vi "Poll FP Change Device List.vi"(8 "Error In":errorcluster, 10 "First call?":bool, 11 "Device List State":T1) -> (0 "Error Out":errorcluster, 3 "Device List State out":T1)   [LabVIEW 2015]
uses:
  Device List State.ctl
  Device/Device.lvclass
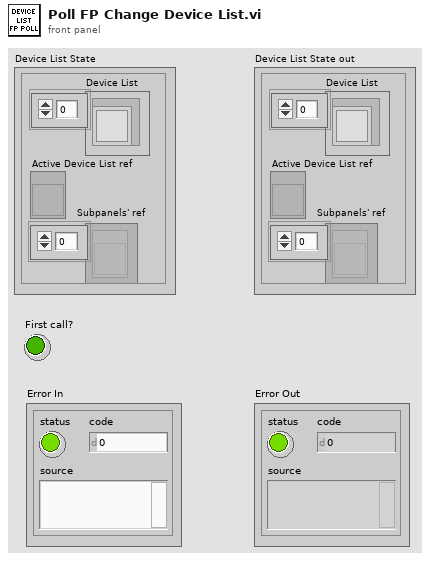
[diagram p1: front panel]
types:
  T1 = typedef "Device List State.ctl" = cluster{"Device List":refnum<class "Device.lvclass">[], "Active Device List ref":refnum<vi>, "Subpanels' ref":refnum<vi>[]}
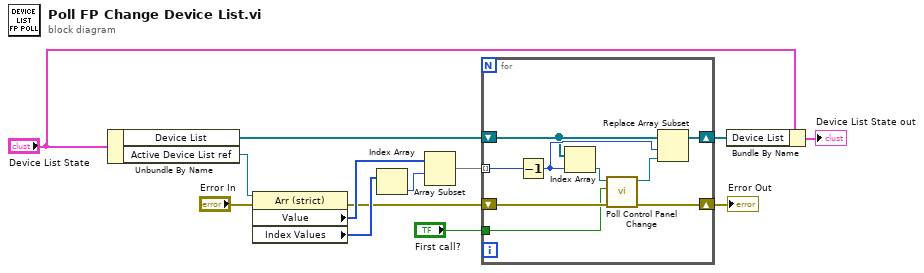
[diagram p0: block diagram]
diagram:
  n1 = Unbundle By Name("Device List State") -> ("Device List"=w7:refnum<class "Device.lvclass">[], "Active Device List ref"=w12:refnum<vi>)
  n2 = property class="Arr (strict)"(reference=w12, error in="Error In") -> (error out=w6:errorcluster, "Value"=w11:u16[], "Index Values"=w9:u32[])  [unwired: 1 out]
  n3 = Index Array(array=w9) -> (element=w10:u32)  [unwired: 1 in]
  n4 = Array Subset(array=w11, index=w10) -> (w8:u16[])  [unwired: 1 in]
  n5 = for {
    tunnel: w8 -> [w22] mode=indexing
    shift-right: [w19] -> w3
    shift-left: w6 -> [w21]
    tunnel: "First call?" -> [w18]
    shift-right: [w14] -> w2
    shift-left: w7 -> [w16]
    n6 = Decrement(x=w22) -> (x-1=w17:u16)
    n7 = Index Array(array=w16, index=w17) -> (element=w20:refnum<class "Device.lvclass">)
    n8 = call "Poll Control Panel Change.vi"("error in (no error)"=w21, "First call?"=w18, "Device"=w20) -> ("error out"=w19:errorcluster, "Device out"=w15:refnum<class "Device.lvclass">)  [unwired: 7 in]
    n9 = Replace Array Subset(array=w16, new element=w15, index=w17) -> (w14:refnum<class "Device.lvclass">[])
  }
  "Error Out" <- w3
  n10 = Bundle By Name(cluster="Device List State", "Device List"=w2) -> (→"Device List State out":T1)
